vi "IL Actor Construct.vi"() -> ()   [LabVIEW 2015]
uses:
  Interlocks/Interlock Bool/Interlock Bool.lvclass
  Interlocks/Interlock Chain/Interlock Chain.lvclass
  Interlocks/Interlock Bool/Interlock Bool.lvclass/Interlock Bool.ctl
  Interlocks/Interlock/Interlock.lvclass/Interlock.ctl
  <vilib>/ActorFramework/Message Enqueuer/Message Enqueuer.lvclass/Message Enqueuer.ctl
  <vilib>/ActorFramework/Stop Msg/Send Emergency Stop.vi
  <vilib>/ActorFramework/Stop Msg/Send Normal Stop.vi
  <vilib>/ActorFramework/Message Enqueuer/Enqueue Critical.vi
  <vilib>/ActorFramework/Message Enqueuer/Enqueue.vi
  <vilib>/ActorFramework/Message Priority Queue/Priority Enqueue.vi
  <vilib>/ActorFramework/Stop Msg/Stop Msg.lvclass
  Interlocks/Interlock/Interlock.lvclass
  Interlocks/IL Action/IL Action.lvclass
  <vilib>/ActorFramework/Actor/Actor.lvclass
panel:
  out "Numeric 2":i32
  out "error out":errorcluster
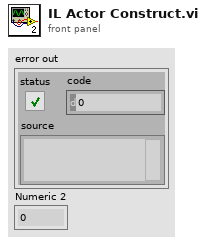
[diagram p1: front panel]
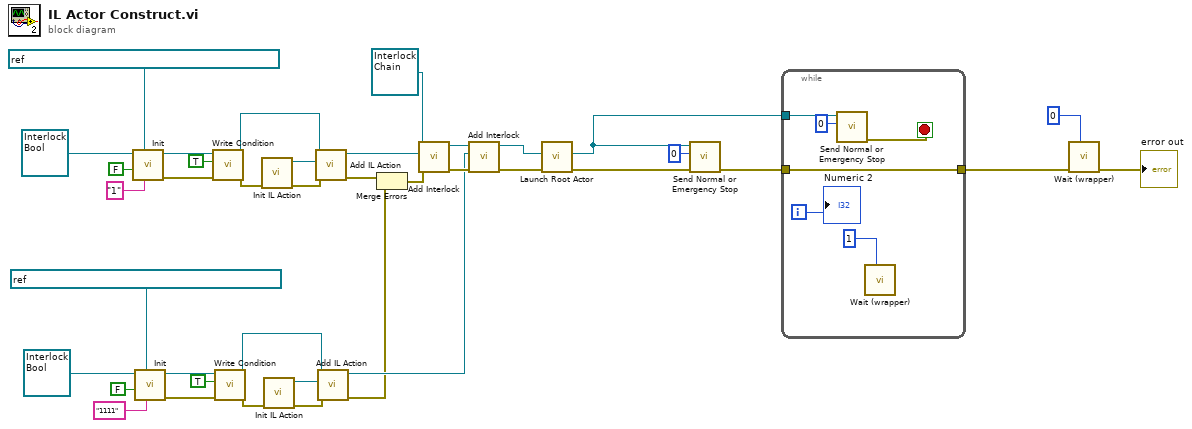
[diagram p0: block diagram]
diagram:
  n1 = call-dynamic "Init.vi"("Name (SHV Name if empty)"="1", "SHV"=refnum<k21> "ni.var.psp://10.2.0.20/AMS Gas SHV/Stop Core" ("shared variable refnum in"), "Stop Self on IL? (T)"=FALSE, "Interlock in"=refnum<class "Interlock Bool.lvclass"> refnum ("Interlocks.lvlib:Interlock Bool.lvclass")) -> ("error out"=w35:errorcluster, "Interlock out"=w37:refnum<class "Interlock Bool.lvclass">)  [unwired: 6 in]
  n2 = call-dynamic "Init.vi"("Name (SHV Name if empty)"="1111", "SHV"=refnum<k21> "ni.var.psp://10.2.0.20/AMS Gas SHV/Stop Core" ("shared variable refnum in"), "Stop Self on IL? (T)"=FALSE, "Interlock in"=refnum<class "Interlock Bool.lvclass"> refnum ("Interlocks.lvlib:Interlock Bool.lvclass")) -> ("error out"=w20:errorcluster, "Interlock out"=w18:refnum<class "Interlock Bool.lvclass">)  [unwired: 6 in]
  n3 = call "Write Condition.vi"("error in (no error)"=w35, "Interlock Condition"=TRUE, "Interlock Bool in"=w37) -> ("error out"=w31:errorcluster, "Interlock Bool out"=w34:refnum<class "Interlock Bool.lvclass">)  [unwired: 7 in]
  n4 = call "Write Condition.vi"("error in (no error)"=w20, "Interlock Condition"=TRUE, "Interlock Bool in"=w18) -> ("error out"=w24:errorcluster, "Interlock Bool out"=w21:refnum<class "Interlock Bool.lvclass">)  [unwired: 7 in]
  n5 = call "Init IL Action.vi"("error in (no error)"=w31) -> ("error out"=w32:errorcluster, "IL Action out"=w33:refnum<class "IL Action.lvclass">)  [unwired: 9 in]
  n6 = call "Init IL Action.vi"("error in (no error)"=w24) -> ("error out"=w23:errorcluster, "IL Action out"=w22:refnum<class "IL Action.lvclass">)  [unwired: 9 in]
  n7 = call "Add IL Action.vi"("error in (no error)"=w32, "IL Action in"=w33, "Interlock in"=w34) -> ("error out"=w8:errorcluster, "Interlock out"=w10:refnum<class "Interlock Bool.lvclass">)  [unwired: 7 in]
  n8 = call "Add IL Action.vi"("error in (no error)"=w23, "IL Action in"=w22, "Interlock in"=w21) -> ("error out"=w6:errorcluster, "Interlock out"=w9:refnum<class "Interlock Bool.lvclass">)  [unwired: 7 in]
  n9 = Merge Errors(w8, w6) -> (w7:errorcluster)
  n10 = call "Add Interlock.vi"("error in (no error)"=w7, "Interlock.lvclass"=w10, "Interlock Chain in"=refnum<class "Interlock Chain.lvclass"> refnum) -> ("error out"=w13:errorcluster, "Interlock Chain out"=w12:refnum<class "Interlock Chain.lvclass">)  [unwired: 7 in]
  n11 = call "Add Interlock.vi"("error in (no error)"=w13, "Interlock.lvclass"=w9, "Interlock Chain in"=w12) -> ("error out"=w5:errorcluster, "Interlock Chain out"=w4:refnum<class "Interlock Chain.lvclass">)  [unwired: 7 in]
  n12 = call <vilib>:"Launch Root Actor.vi"("error in (no error)"=w5, "Actor"=w4) -> ("error out"=w30:errorcluster, "Actor's Enqueuer"=w1:refnum<class "Message Enqueuer.lvclass">)  [unwired: 8 in]
  n13 = call <vilib>:"Send Normal or Emergency Stop.vi"("error in (no error)"=w30, "final error code"=0, "Message Enqueuer"=w1) -> ("error out"=w3:errorcluster)  [unwired: 8 in]
  n14 = while {
    tunnel: w3 -> [w45]
    tunnel: [w45] -> w2
    tunnel: w1 -> [w43]
    i -> [w44]
    stop <- w41 stop-if-true
    n15 = call <vilib>:"Send Normal or Emergency Stop.vi"("final error code"=0, "Message Enqueuer"=w43) -> ("error out"=w41:errorcluster)  [unwired: 9 in]
    n16 = call "Wait (wrapper).vi"("milliseconds to wait (200)"=u32 1) -> ()  [unwired: 10 in, 1 out]
    "Numeric 2" <- w44
  }
  n17 = call "Wait (wrapper).vi"("milliseconds to wait (200)"=u32 0, "error in (no error)"=w2) -> ("error out"=→"error out":errorcluster)  [unwired: 9 in]
